vi "Write Asserted Object Name.vi"(8 "error in (no error)":errorcluster, 10 "Asserted Object Name":string, 11 "Assertion Step in":refnum<class "Assertion Step.lvclass">) -> (0 "error out":errorcluster, 3 "Assertion Step out":refnum<class "Assertion Step.lvclass">)   [LabVIEW 2020, in "MacroAssert.lvlib" / "Assertion Step.lvclass"]
uses:
  Assertion Step.lvclass
  Assertion Step.lvclass/Assertion Step.ctl
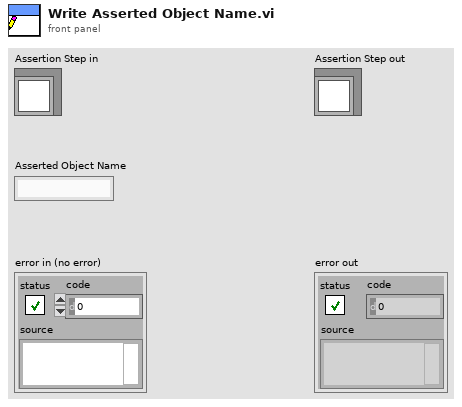
[diagram p1: front panel]
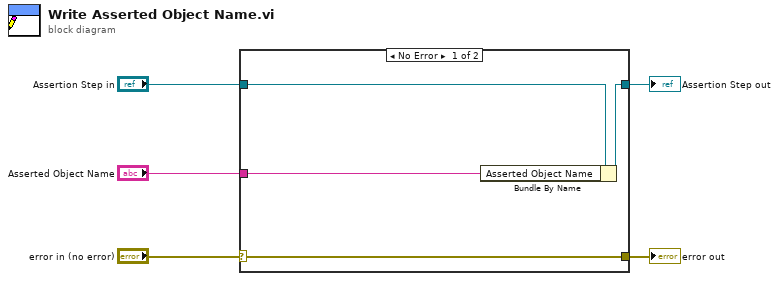
[diagram p0: block diagram]
diagram:
  n1 = case shown="No Error" "error in (no error)" {
    selector: "error in (no error)" -> [w9 w10]
    tunnel: [w9 w10] -> w4
    tunnel: [w7 w11] -> w2
    tunnel: "Assertion Step in" -> [w8 w11]
    tunnel: "Asserted Object Name" -> [w6 _]
    frame No Error {
      n2 = Bundle By Name(cluster=w8, "Asserted Object Name"=w6) -> (w7:refnum<class "Assertion Step.lvclass">)
    }
    frame Error {
    }
  }
  "error out" <- w4
  "Assertion Step out" <- w2
